vi "uMsg Rename CMD.vi"(8 "error in (no error)":errorcluster, 10 "New CMD":string, 11 "uMsg in":refnum<class "uMsg.lvclass">) -> (0 "error out":errorcluster, 3 "uMsg out":refnum<class "uMsg.lvclass">)   [LabVIEW 2023, in "uLib.lvlib" / "uMsg.lvclass"]
doc: "Change the command string."
uses:
  uMsg.lvclass
  uMsg.lvclass/uMsg.ctl
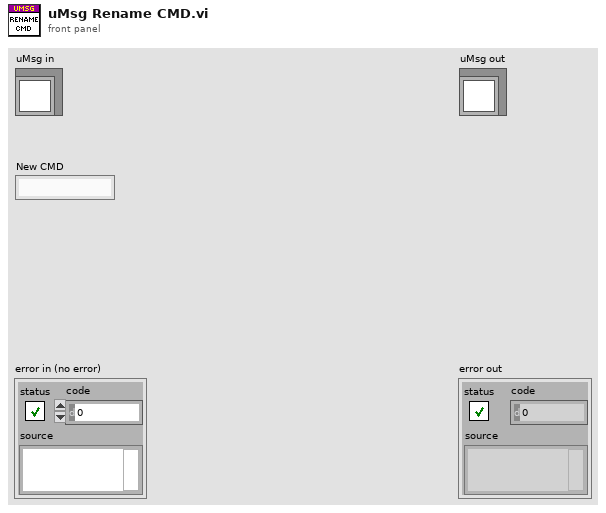
[diagram p1: front panel]
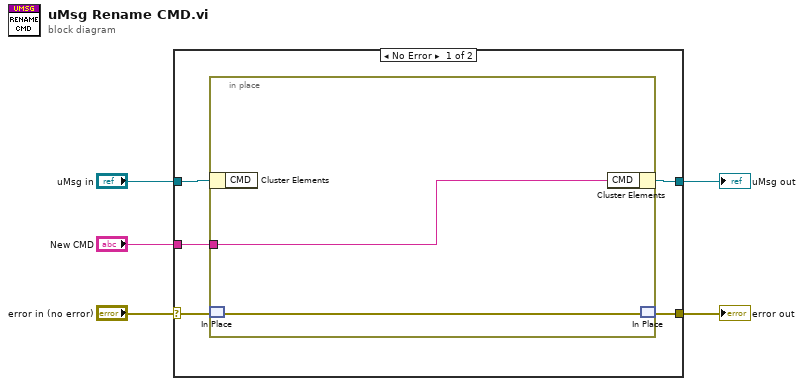
[diagram p0: block diagram]
diagram:
  n1 = case shown="No Error" "error in (no error)" {
    selector: "error in (no error)" -> [w8 w14]
    tunnel: [w7 w14] -> w5
    tunnel: [w10 w13] -> w4
    tunnel: "uMsg in" -> [w9 w13]
    tunnel: "New CMD" -> [w6 _]
    frame No Error {
      n2 = in-place {
        in-place-border: w6 -> [w11]
        n3 = in-place-cluster #1(w9) -> ()  [unwired: 1 out]
        n4 = in-place-match #2(w8) -> (w12:errorcluster)
        n5 = in-place-cluster #1("CMD"=w11) -> (w10:refnum<class "uMsg.lvclass">)
        n6 = in-place-match #2(w12) -> (w7:errorcluster)
      }
    }
    frame Error {
    }
  }
  "error out" <- w5
  "uMsg out" <- w4
